vi "Ok_search.vi"(1 "Display":string="SEGGER J-Link Commander V7.86f (Compiled Mar 29 2023 16:41:57)\nDLL version V7.86f, compiled Mar 29 2023 16:39:17\n\n\nJ-Link Command File read successfully.\nProcessing script file...\nJ-Link>r\nJ-Link connection not established yet but required for command.\nConnecting to J-Link via USB...O.K.\nFirmware: J-Link V11 compiled Sep  3 2024 10:40:48\nHardware version: V11.00\nJ-Link uptime (since boot): 0d 00h 06m 07s\nS/N: 51020673\nLicense(s): GDB\nUSB speed mode: High speed (480 MBit/s)\nVTref=3.019V\nTarget connection not established yet but required for command.\nDevice \"R7FA4E10D\" selected.\n\n\nConnecting to target via SWD\nConfigTargetSettings() start\nConfiguring FlashDLNoRMWThreshold=0x200 in order to make sure that option bytes programming is done via read-modify-write\nConfigTargetSettings() end - Took 10us\nInitTarget() start\nSWD selected. Executing JTAG -> SWD switching sequence.\nDAP initialized successfully.\nDetermining TrustZone configuration...\n  Secure Debug: Enabled (SSD)\nDetermining currently configured transfer type by reading the AHB-AP CSW register.\n  --> Correct transfer type configured. Done.\nInitTarget() end - Took 6.07ms\nFound SW-DP with ID 0x6BA02477\nDPIDR: 0x6BA02477\nCoreSight SoC-400 or earlier\nScanning AP map to find all available APs\nAP[2]: Stopped AP scan as end of AP map has been reached\nAP[0]: AHB-AP (IDR: 0x84770001)\nAP[1]: APB-AP (IDR: 0x54770002)\nIterating through AP map to find AHB-AP to use\nAP[0]: Core found\nAP[0]: AHB-AP ROM base: 0xE00FE000\nCPUID register: 0x410FD214. Implementer code: 0x41 (ARM)\nFeature set: Mainline\nCache: No cache\nFound Cortex-M33 r0p4, Little endian.\nFPUnit: 8 code (BP) slots and 0 literal slots\nSecurity extension: implemented\nSecure debug: enabled\nCoreSight components:\nROMTbl[0] @ E00FE000\n[0][0]: E0044000 CID B105900D PID 005BB906 DEVARCH 00000000 DEVTYPE 14 CTI (?)\n[0][1]: E0047000 CID B105900D PID 003BB908 DEVARCH 00000000 DEVTYPE 12 CSTF\n[0][2]: E0048000 CID B105900D PID 001BB961 DEVARCH 00000000 DEVTYPE 21 ETB\n[0][3]: E0049000 CID B105F00D PID 001BB101 TSG\n[0][4]: E0040000 CID B105900D PID 000BBD21 DEVARCH 00000000 DEVTYPE 11 TPIU\n[0][5]: E00FF000 CID B105100D PID 000BB4C9 ROM Table\nROMTbl[1] @ E00FF000\n[1][0]: E000E000 CID B105900D PID 000BBD21 DEVARCH 47702A04 DEVTYPE 00 Cortex-M33\n[1][1]: E0001000 CID B105900D PID 000BBD21 DEVARCH 47701A02 DEVTYPE 00 DWT\n[1][2]: E0002000 CID B105900D PID 000BBD21 DEVARCH 47701A03 DEVTYPE 00 FPB\n[1][3]: E0000000 CID B105900D PID 000BBD21 DEVARCH 47701A01 DEVTYPE 43 ITM\n[1][5]: E0041000 CID B105900D PID 002BBD21 DEVARCH 47724A13 DEVTYPE 13 ETM\n[1][6]: E0042000 CID B105900D PID 000BBD21 DEVARCH 47701A14 DEVTYPE 14 CSS600-CTI\nMemory zones:\n  Zone: \"Default\" Description: Default access mode\nCortex-M33 identified.\nReset delay: 0 ms\nReset type NORMAL: Resets core & peripherals via SYSRESETREQ & VECTRESET bit.\nReset: ARMv8M core with Security Extension enabled detected.\nReset: Halt core after reset via DEMCR.VC_CORERESET.\nReset: Reset device via AIRCR.SYSRESETREQ.\nJ-Link>h\nPC = 00008158, CycleCnt = 00000000\nR0 = 00000000, R1 = 00000000, R2 = 00000000, R3 = 00000000\nR4 = 00000000, R5 = 00000000, R6 = 00000000, R7 = 00000000\nR8 = 0001E848, R9 = 00000000, R10= A5A5A5A5, R11= A5A5A5A5\nR12= A5A5A5A5\nSP(R13)= 20004BD8, MSP= 20004BD8, PSP= 00000000, R14(LR) = FFFFFFFF\nXPSR = F9000000: APSR = NZCVQ, EPSR = 01000000, IPSR = 000 (NoException)\nCFBP = 00000000, CONTROL = 00, FAULTMASK = 00, BASEPRI = 00, PRIMASK = 00\nMSPLIM = 00000000\nPSPLIM = 00000000\n\nSecurity extension regs:\nMSP_S = 20004BD8, MSP_NS = 00000000\nMSPLIM_S = 00000000, MSPLIM_NS = 00000000\nPSP_S = 00000000, PSP_NS = 2E56C7C8\nPSPLIM_S = 00000000, PSPLIM_NS = 00000000\nCONTROL_S  = 00, FAULTMASK_S  = 00, BASEPRI_S  = 00, PRIMASK_S  = 00\nCONTROL_NS = 00, FAULTMASK_NS = 00, BASEPRI_NS = 00, PRIMASK_NS = 00\n\nFPS0 = 00000000, FPS1 = 00000000, FPS2 = 00000000, FPS3 = 00000000\nFPS4 = 00000000, FPS5 = 00000000, FPS6 = 00000000, FPS7 = 00000000\nFPS8 = 00000000, FPS9 = 00000000, FPS10= 00000000, FPS11= 00000000\nFPS12= 00000000, FPS13= 00000000, FPS14= 00000000, FPS15= 00000000\nFPS16= 00000000, FPS17= 00000000, FPS18= 00000000, FPS19= 00000000\nFPS20= 00000000, FPS21= 00000000, FPS22= 00000000, FPS23= 00000000\nFPS24= 00000000, FPS25= 00000000, FPS26= 00000000, FPS27= 00000000\nFPS28= 00000000, FPS29= 00000000, FPS30= 00000000, FPS31= 00000000\nFPSCR= 00000000\nJ-Link>erase\nNo address range specified, 'Erase Chip' will be executed\n'erase': Performing implicit reset & halt of MCU.\nReset: ARMv8M core with Security Extension enabled detected.\nReset: Halt core after reset via DEMCR.VC_CORERESET.\nReset: Reset device via AIRCR.SYSRESETREQ.\nErasing device...\nJ-Link: Flash download: Only internal flash banks will be erased.\nTo enable erasing of other flash banks like QSPI or CFI, it needs to be enabled via \"exec EnableEraseAllFlashBanks\"\nJ-Link: Flash download: Total time needed: 0.719s (Prepare: 0.329s, Compare: 0.000s, Erase: 0.335s, Program: 0.000s, Verify: 0.000s, Restore: 0.054s)\nJ-Link: Flash download: Total time needed: 1.478s (Prepare: 0.266s, Compare: 0.000s, Erase: 1.070s, Program: 0.000s, Verify: 0.000s, Restore: 0.140s)\nJ-Link: Flash download: Total time needed: 0.431s (Prepare: 0.186s, Compare: 0.000s, Erase: 0.189s, Program: 0.000s, Verify: 0.000s, Restore: 0.055s)\nErasing done.\nJ-Link>loadfile \"C:\\Users\\A. Halstesd Evander\\Documents\\DTU_Manual_Flash\\Info\\Configuration\\app.hex\"\n'loadfile': Performing implicit reset & halt of MCU.\nReset: ARMv8M core with Security Extension enabled detected.\nReset: Halt core after reset via DEMCR.VC_CORERESET.\nReset: Reset device via AIRCR.SYSRESETREQ.\nDownloading file [C:\\Users\\A. Halstesd Evander\\Documents\\DTU_Manual_Flash\\Info\\Configuration\\app.hex]...\nJ-Link: Flash download: Bank 0 @ 0x0100A100: 2 ranges affected (32 bytes)\nJ-Link: Flash download: Total: 0.368s (Prepare: 0.176s, Compare: 0.106s, Erase: 0.000s, Program & Verify: 0.029s, Restore: 0.056s)\nJ-Link: Flash download: Program & Verify speed: 1 KB/s\nJ-Link: Flash download: Bank 1 @ 0x00000000: 2 ranges affected (172032 bytes)\nJ-Link: Flash download: Total: 2.505s (Prepare: 0.268s, Compare: 0.065s, Erase: 0.000s, Program & Verify: 2.024s, Restore: 0.146s)\nJ-Link: Flash download: Program & Verify speed: 82 KB/s\nO.K.\nJ-Link>r\nReset delay: 0 ms\nReset type NORMAL: Resets core & peripherals via SYSRESETREQ & VECTRESET bit.\nReset: ARMv8M core with Security Extension enabled detected.\nReset: Halt core after reset via DEMCR.VC_CORERESET.\nReset: Reset device via AIRCR.SYSRESETREQ.\nJ-Link>g\nJ-Link>exit\n\nScript processing completed.\n\nSerial Number: 51020673 \n") -> (0 "index of element":i32)   [LabVIEW 2024, in "MCU_Flashing.lvlib"]
uses:
  MCU_Flashing.lvlib
panel:
  out "array":string[](array[string])
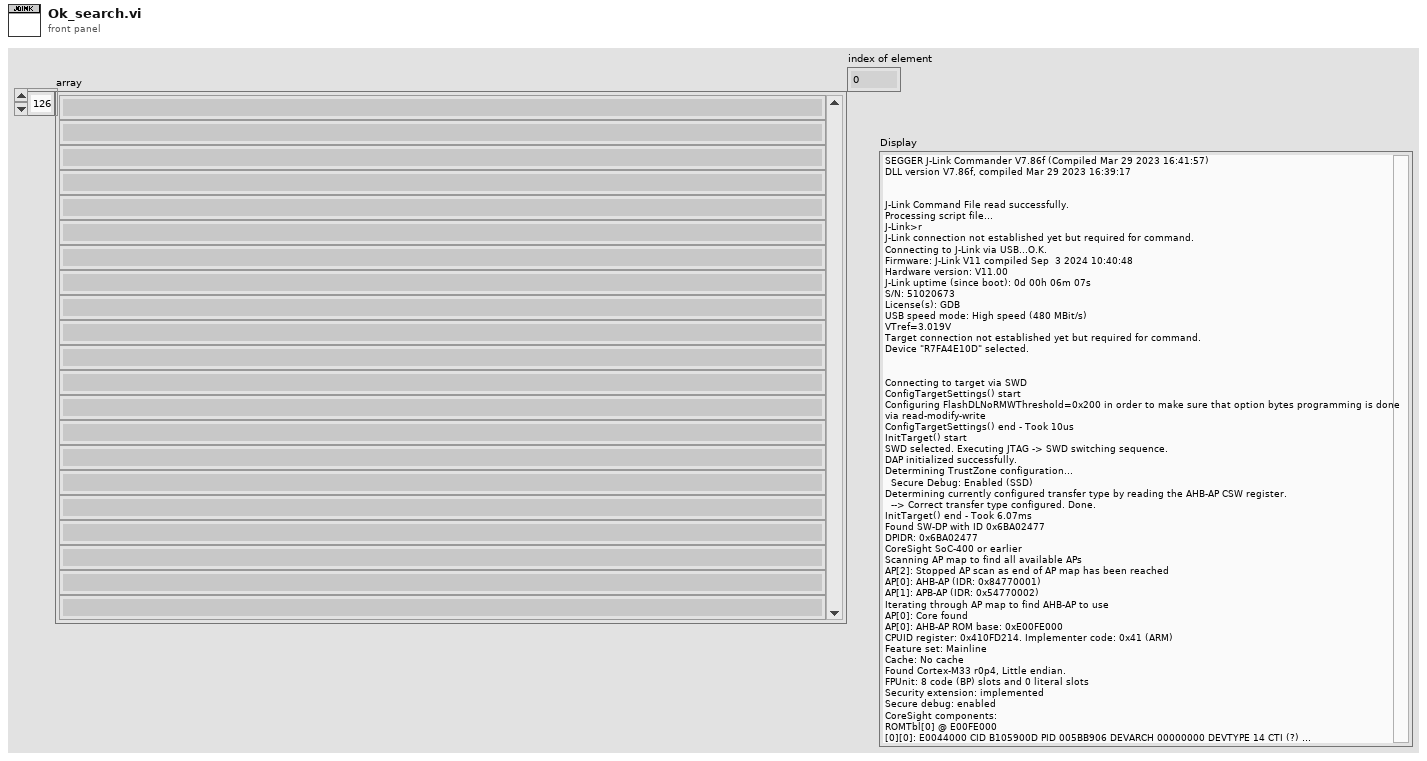
[diagram p1: front panel]
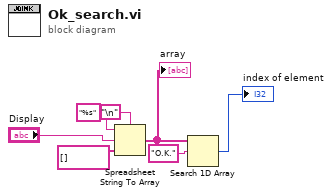
[diagram p0: block diagram]
diagram:
  n1 = Spreadsheet String To Array(delimiter (Tab)="\n", format string="%s", spreadsheet string="Display", array type (2D Dbl)=string[] []) -> (array=w3:string[])
  "array" <- w3
  n2 = Search 1D Array(1D array=w3, element="O.K.") -> (index of element=→"index of element":i32)  [unwired: 1 in]
